vi "WriteDM.vi"(0 "reference in":refnum<k7>, 1 "nDevId":i32, 2 "MultiDM  Mapping":i32[](array[numeric]), 3 "Voltage Array in":u16[](array[numeric]), 4 "error in":errorcluster) -> (5 "reference out":refnum<k7>, 7 "error out":errorcluster)   [LabVIEW 2014]
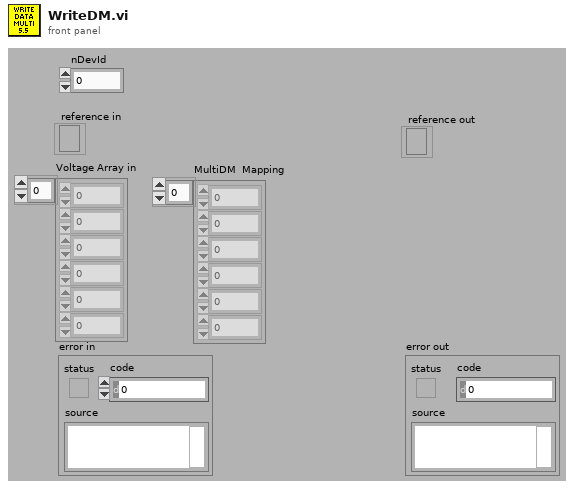
[diagram p1: front panel]
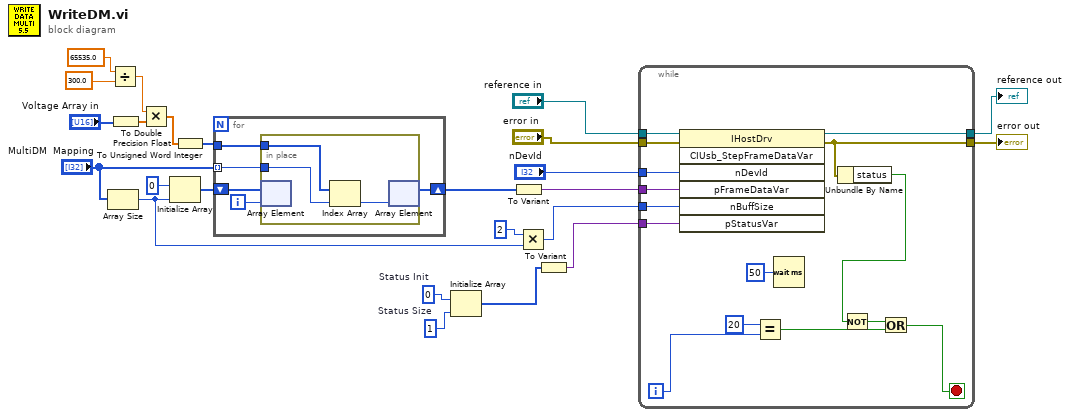
[diagram p0: block diagram]
diagram:
  w9 = 1  # Status Size
  w8 = 0  # Status Init
  n1 = Array Size(array="MultiDM  Mapping") -> (size(s)=w3:i32)
  n2 = Divide(x=65535.0 ("y"), y=300.0 ("x")) -> (x/y=w4:dbl)
  n3 = To Double Precision Float(number="Voltage Array in") -> (double precision float=w5:dbl[])
  n4 = Multiply(x=w4, y=w5) -> (x*y=w19:dbl[])
  n5 = Initialize Array(u16 0 ("element"), w3) -> (w17:u16[])
  n6 = To Unsigned Word Integer(number=w19) -> (unsigned 16bit integer=w15:u16[])
  n7 = for {
    shift-right: [w27] -> w14
    shift-left: w17 -> [w29]
    tunnel: "MultiDM  Mapping" -> [w25] mode=indexing
    tunnel: w15 -> [w28]
    i -> [w26]
    n8 = in-place {
      in-place-border: w28 -> [w31]
      in-place-border: w25 -> [w32]
      n9 = in-place-array #1(w29, w26) -> ()  [unwired: 1 out]
      n10 = Index Array(array=w31, index=w32) -> (element=w30:u16)
      n11 = in-place-array #1(w30) -> (w27:u16[])  [unwired: 1 out]
    }
  }
  n12 = Initialize Array "Initialize Array"(w8, w9) -> (w7:i32[])
  n13 = To Variant(anything=w14) -> (Variant=w22:variant)
  n14 = Multiply(x=2, y=w3) -> (x*y=w1:i32)
  n15 = To Variant(anything=w7) -> (Variant=w6:variant)
  n16 = while {
    tunnel: [w47] -> w24
    tunnel: [w40] -> w23
    tunnel: w22 -> [w46]
    tunnel: "error in" -> [w45]
    tunnel: "reference in" -> [w44]
    tunnel: "nDevId" -> [w43]
    tunnel: w6 -> [w42]
    tunnel: w1 -> [w41]
    i -> [w39]
    stop <- w34 stop-if-true
    n17 = invoke class="IHostDrv" method="CIUsb_StepFrameDataVar"(reference=w44, error in=w45, "nDevId"=w43, "pFrameDataVar"=w46, "nBuffSize"=w41, "pStatusVar"=w42) -> (reference out=w47:refnum<k7>, error out=w40:errorcluster)  [unwired: 1 in, 5 out]
    n18 = Equal?(x=20, y=w39) -> (x = y?=w37:bool)
    n19 = Wait (ms)(milliseconds to wait=u32 50) -> ()  [unwired: 1 out]
    n20 = Unbundle By Name(w40) -> ("status"=w36:bool)
    n21 = Not(x=w36) -> (.not. x?=w35:bool)
    n22 = Or(x=w35, y=w37) -> (x .or. y?=w34:bool)
  }
  "error out" <- w23
  "reference out" <- w24
